vi "Multiply Gains.vi"(1 "Other Gain":dbl[](array[numeric]), 2 "Gain":dbl[](array[numeric])) -> (0 "Gain x Other Gain":dbl[](array[numeric]))   [LabVIEW 2016, in "Control Experiment.lvclass"]
uses:
  Control Experiment.lvclass
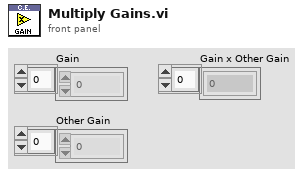
[diagram p1: front panel]
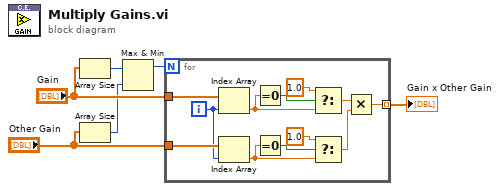
[diagram p0: block diagram]
diagram:
  n1 = Array Size(array="Gain") -> (size(s)=w3:i32)
  n2 = Array Size(array="Other Gain") -> (size(s)=w2:i32)
  n3 = Max & Min(x=w3, y=w2) -> (max(x,y)=w1:i32)  [unwired: 1 out]
  n4 = for {
    N: w1 -> [_]
    tunnel: "Gain" -> [w12]
    tunnel: "Other Gain" -> [w17]
    tunnel: [w18] -> w6 mode=indexing
    i -> [w11]
    n5 = Index Array(array=w12, index=w11) -> (element=w8:dbl)
    n6 = Index Array(array=w17, index=w11) -> (element=w14:dbl)
    n7 = Equal To 0?(x=w8) -> (x = 0?=w9:bool)
    n8 = Equal To 0?(x=w14) -> (x = 0?=w16:bool)
    n9 = Select(t=1.0, s=w9, f=w8) -> (s? t:f=w7:dbl)
    n10 = Select(t=1.0, s=w16, f=w14) -> (s? t:f=w15:dbl)
    n11 = Multiply(x=w7, y=w15) -> (x*y=w18:dbl)
  }
  "Gain x Other Gain" <- w6
